vi "Day 19-Parse Data.vi"(11 "Data in":string[](array[string])) -> (3 "Beacon Coordinate by Scanner":cluster{i32[][]}[](array[cluster]))   [LabVIEW 2021]
uses:
  <vilib>/regexp/Match Regular Expression.xnode
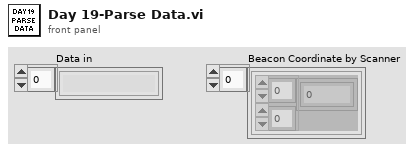
[diagram p1: front panel]
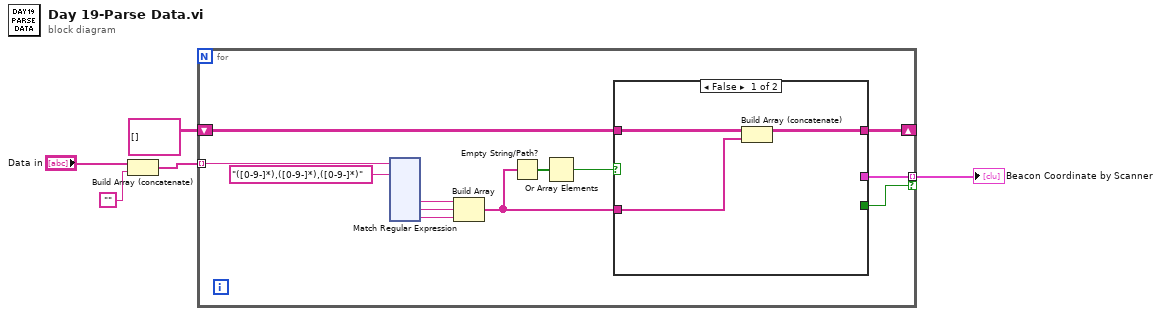
[diagram p0: block diagram]
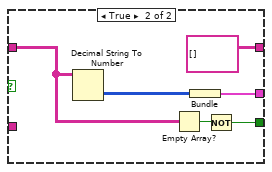
[diagram p2: hidden frame]
diagram:
  n1 = Build Array (concatenate)("Data in", "") -> (w4:string[])
  n2 = for {
    tunnel: w4 -> [w17] mode=indexing
    shift-right: [w11] -> _
    shift-left: string[][] [] -> [w12]
    tunnel: [w10] -> w3 mode=indexing if=w9
    n3 = xnode "Match Regular Expression"("input string"=w17, "regular expression"="([0-9-]*),([0-9-]*),([0-9-]*)") -> ("submatch 1"=w15:string, "submatch 2"=w14:string, "submatch 3"=w13:string)  [unwired: 4 in, 5 out]
    n4 = Build Array(w15, w14, w13) -> (w8:string[])
    n5 = Empty String/Path?(string/path=w8) -> (empty?=w7:bool[])
    n6 = Or Array Elements(Boolean array=w7) -> (logical OR=w6:bool)
    n7 = case shown="False" w6 {
      tunnel: w8 -> [w20 _]
      tunnel: w12 -> [w19 w21]
      tunnel: [w18 string[][] []] -> w11
      tunnel: [_ w23] -> w10
      tunnel: [_ w24] -> w9
      frame False {
        n8 = Build Array (concatenate)(w19, w20) -> (w18:string[][])
      }
      frame True {
        n9 = Decimal String To Number(string=w21) -> (number=w22:i32[][])  [unwired: 2 in, 1 out]
        n10 = Empty Array?(array=w21) -> (empty?=w25:bool)
        n11 = Bundle(w22) -> (w23:cluster{i32[][]})  [unwired: 1 in]
        n12 = Not(x=w25) -> (.not. x?=w24:bool)
      }
    }
  }
  "Beacon Coordinate by Scanner" <- w3
